vi "Cipher.vi"(5 "Key(input)":u32[](array[numeric])=[64, 226, 1, 0, 21, 21, 21, 21, 0, 0, 0, 0, 0, 0, 0, 0], 9 "ExpandedKey(w)1D":u32[](array[numeric]), 11 "error in":errorcluster) -> (8 "Cypher Output":u16[](array[numeric]), 15 "error out":errorcluster)   [LabVIEW 2012, in "Advanced Encryption Standard (AES).lvlib"]
doc: "The AES cipher is specified as a number of repetitions of transformation rounds that convert the input plaintext into the final output of ciphertext. Each round consists of several processing steps, including one that depends on the encryption key.\n\n<inline>"
uses:
  Advanced Encryption Standard (AES).lvlib
  Controls and Typedefs/Cipher Phases Enum (Typedef).ctl
panel:
  in  "Nb":i32=4
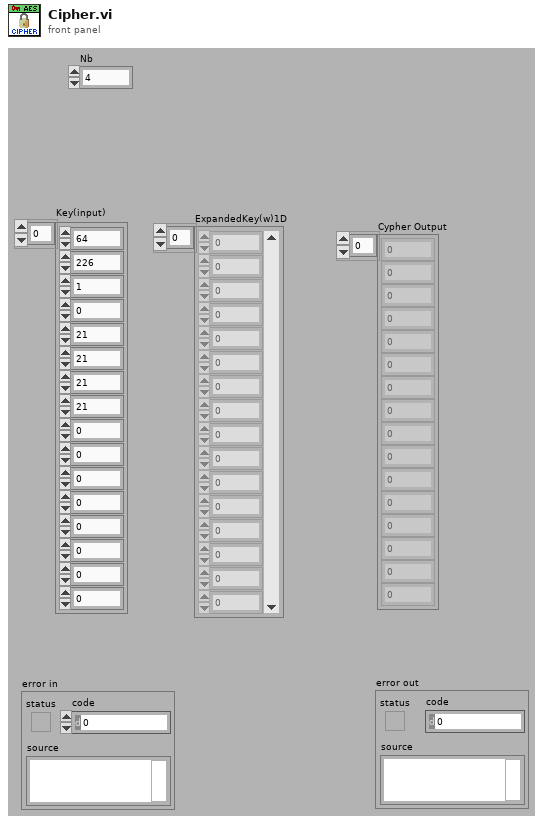
[diagram p1: front panel]
types:
  T1 = typedef "Cipher Phases Enum (Typedef).ctl" = enum16{"Init", "Mix rows"}
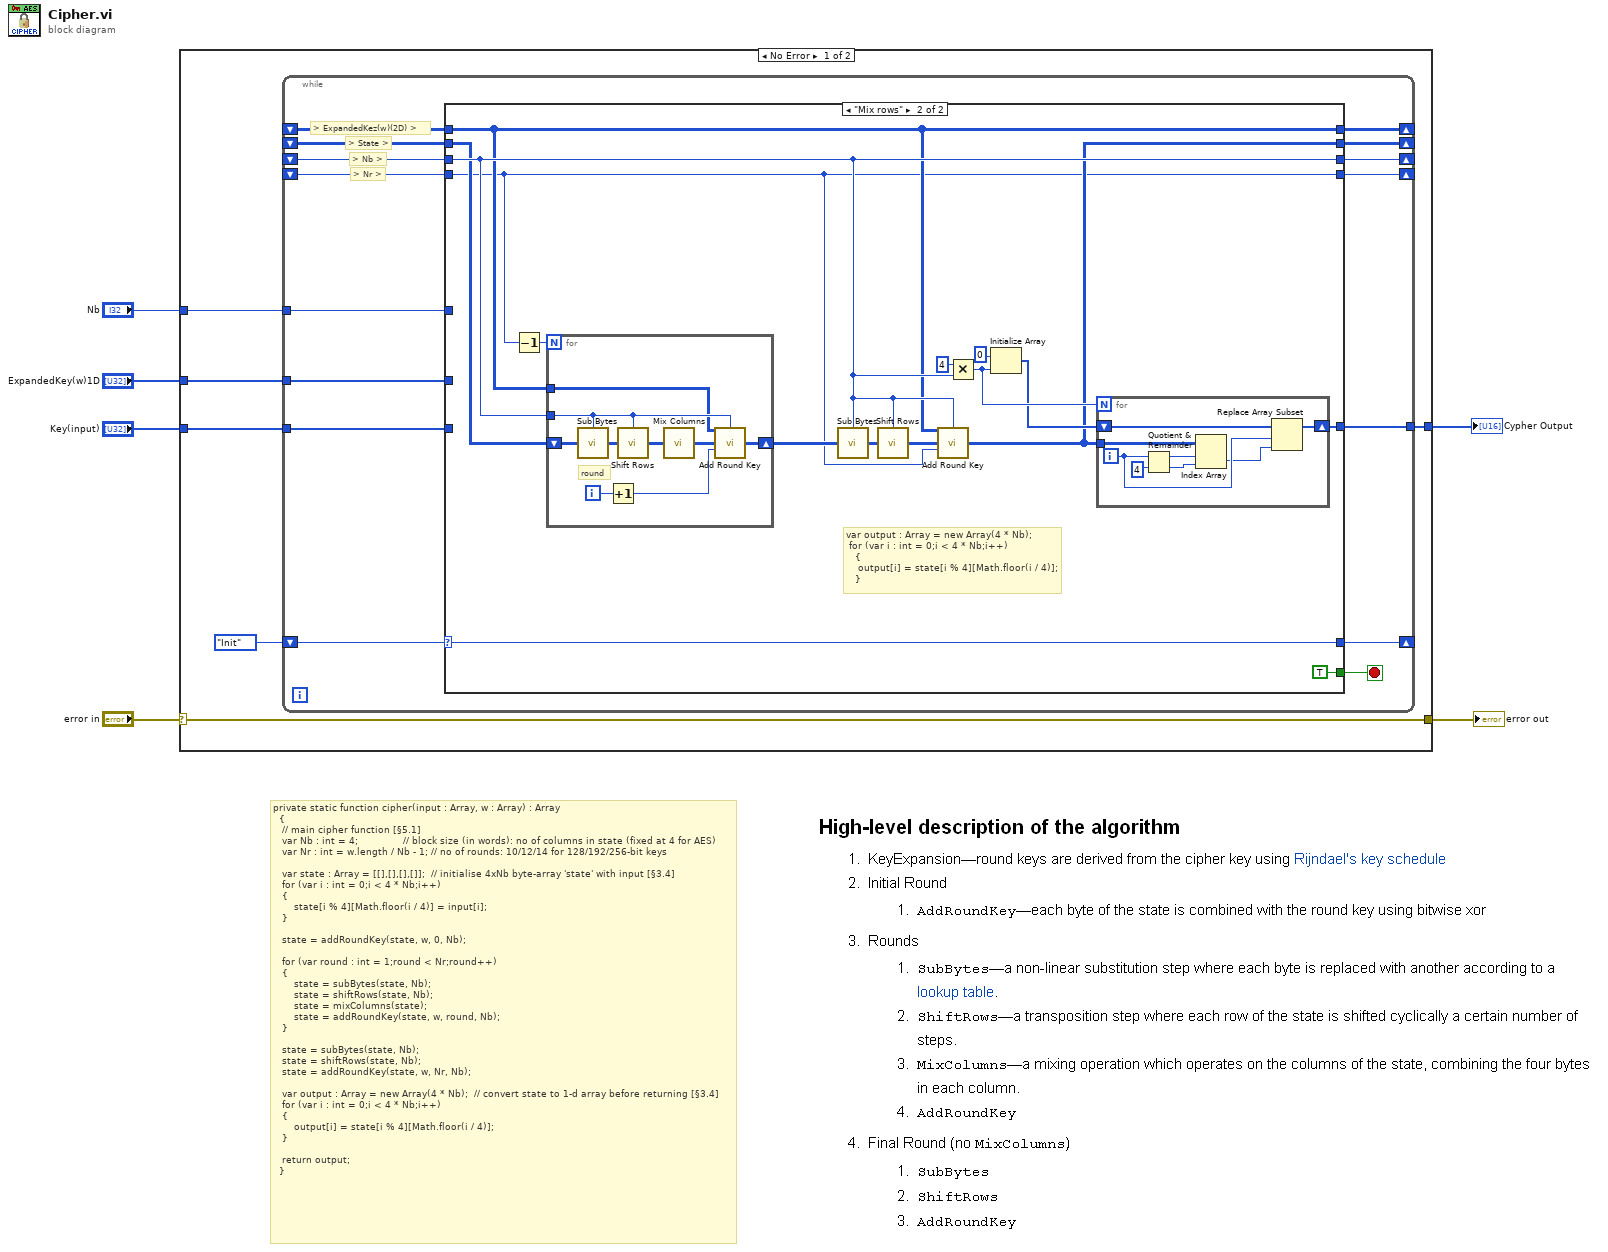
[diagram p0: block diagram]
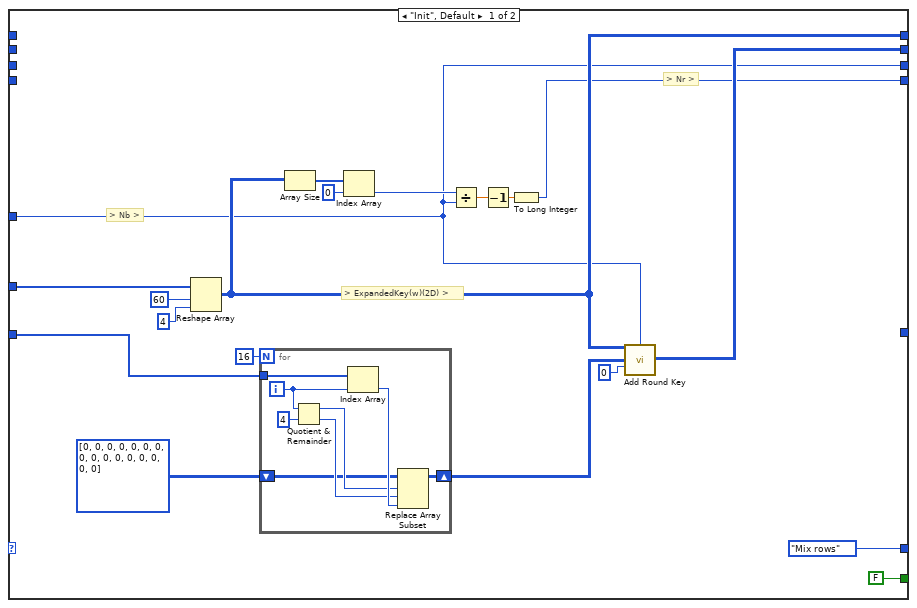
[diagram p2: hidden frame]
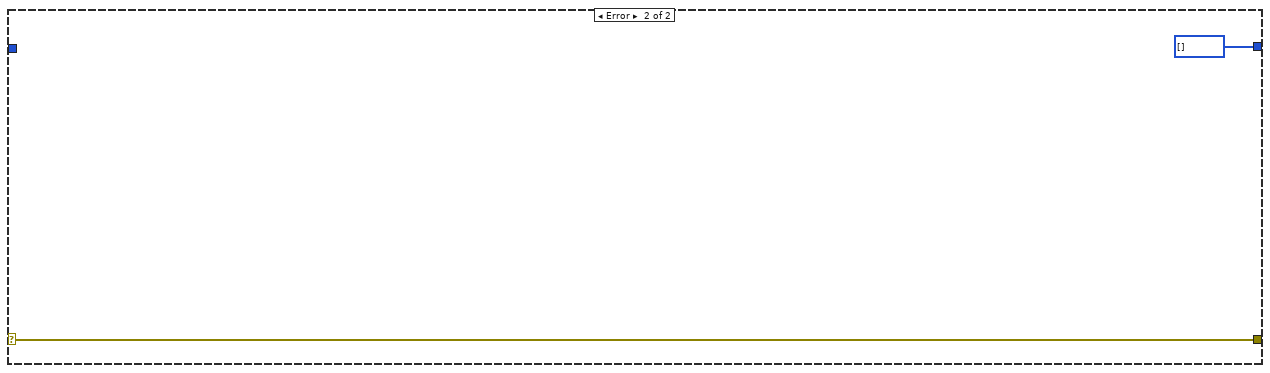
[diagram p3: hidden frame]
diagram:
  # "private static function cipher(input : Array, w : Array) : Array \n\t\t{    \n\t\t\t// main cipher function [§5.1]\n\t\t\tvar Nb : int = 4;               // block size (in words): no of columns in state (fixed at 4 for AES)\n\t\t\tvar Nr : int = w.length / Nb - 1; // no of rounds: 10/12/14 for 128/192/256-bit keys\n\n\t\t\tvar state : Array = [[],[],[],[]];  // initialise 4xNb byte-array 'state' with input [§3.4]\n\t\t\tfor (var i : int = 0;i < 4 * Nb;i++) \n\t\t\t{\n\t\t\t\t   state[i % 4][Math.floor(i / 4)] = input[i];\n\t\t\t}\n\t\t\t\n\t\t\tstate = addRoundKey(state, w, 0, Nb);\n\t\t\t\n\t\t\tfor (var round : int = 1;round < Nr;round++) \n\t\t\t{\n\t\t\t   \tstate = subBytes(state, Nb);\n\t\t   \t\tstate = shiftRows(state, Nb);\n\t\t   \t\tstate = mixColumns(state);\n\t\t   \t\tstate = addRoundKey(state, w, round, Nb);\n\t\t\t}\n\t\t\t\n\t\t\tstate = subBytes(state, Nb);\n\t\t\tstate = shiftRows(state, Nb);\n\t\t\tstate = addRoundKey(state, w, Nr, Nb);\n\t\t\t\n\t\t\tvar output : Array = new Array(4 * Nb);  // convert state to 1-d array before returning [§3.4]\n\t\t\tfor (var i : int = 0;i < 4 * Nb;i++)\n   {\n       output[i] = state[i % 4][Math.floor(i / 4)];\n\t\t\t}\n\n\t\t\treturn output;\n\t\t}"
  n1 = case shown="No Error" "error in" {
    selector: "error in" -> [w7 w89]
    tunnel: [w7 w89] -> w5
    tunnel: "ExpandedKey(w)1D" -> [w11 _]
    tunnel: "Key(input)" -> [w10 _]
    tunnel: [w9 u16[] []] -> w2
    tunnel: "Nb" -> [w8 _]
    frame No Error {
      n2 = while {
        shift-right: [w15] -> _
        shift-left: Cipher_Phases_Enum_(Typedef)."Init" ("Cipher Phases") -> [w27]
        tunnel: w11 -> [w26]
        tunnel: w10 -> [w25]
        shift-right: [w24] -> _
        shift-left: _ -> [w23]
        shift-right: [w22] -> _
        shift-left: _ -> [w21]
        shift-right: [w20] -> _
        shift-left: _ -> [w19]
        shift-right: [w18] -> _
        shift-left: _ -> [w17]
        tunnel: [w16] -> w9
        tunnel: w8 -> [w13]
        stop <- w14 stop-if-true
        # "> Nr >"
        # "> Nb >"
        # "> State >"
        # "> ExpandedKez(w)(2D) >"
        n3 = case shown="\"Mix rows\"" w27 {
          selector: w27 -> [_ w55]
          tunnel: w26 -> [w40 _]
          tunnel: w25 -> [w38 _]
          tunnel: [w36 w63] -> w24
          tunnel: w23 -> [_ w63]
          tunnel: [w35 w57] -> w22
          tunnel: w21 -> [_ w58]
          tunnel: [w30 w64] -> w20
          tunnel: w19 -> [_ w64]
          tunnel: [w33 w56] -> w18
          tunnel: w17 -> [_ w56]
          tunnel: [_ w60] -> w16
          tunnel: [Cipher_Phases_Enum_(Typedef)."Mix rows" ("Cipher Phases") w55] -> w15
          tunnel: [FALSE TRUE] -> w14
          tunnel: w13 -> [w30 _]
          frame "Init", Default {
            # "> Nb >"
            # "> ExpandedKey(w)(2D) >"
            # "> Nr >"
            n4 = Reshape Array(w40, 60 ("dimension size"), 4 ("dimension size")) -> (w36:u32[][])
            n5 = for {
              N: 16 -> [_]
              tunnel: w38 -> [w50]
              shift-right: [w48] -> w37
              shift-left: u16[][] [[0, 0, 0, 0], [0, 0, 0, 0], [0, 0, 0, 0], [0, 0, 0, 0]] ("State.Out") -> [w49]
              i -> [w47]
              n6 = Quotient & Remainder(x=w47, y=4) -> (x-y*floor(x/y)=w52:i32, floor(x/y)=w51:i32)
              n7 = Index Array(array=w50, index=w47) -> (element=w53:u32)
              n8 = Replace Array Subset(array=w49, new element=w53, index (row)=w52, index (col)=w51) -> (w48:u16[][])
            }
            n9 = Array Size(array=w36) -> (size(s)=w41:i32[])
            n10 = Index Array(array=w41, index=0) -> (element=w44:i32)
            n11 = Divide(x=w44, y=w30) -> (x/y=w43:dbl)
            n12 = Decrement(x=w43) -> (x-1=w34:dbl)
            n13 = To Long Integer(number=w34) -> (32bit integer=w33:i32)
            n14 = call "Add Round Key.vi"("ExpandedKey(w)"=w36, "Nb"=w30, "State.In"=w37, "rnd (0)"=0) -> ("State.Out"=w35:u16[][])  [unwired: 10 in, 1 out]
          }
          frame "Mix rows" {
            # "var output : Array = new Array(4 * Nb); \n\tfor (var i : int = 0;i < 4 * Nb;i++)\n   {\n    output[i] = state[i % 4][Math.floor(i / 4)];\n\t\t\t}"
            n15 = Decrement(x=w56) -> (x-1=w70:i32)
            n16 = for {
              N: w70 -> [_]
              shift-right: [w82] -> w65
              shift-left: w58 -> [w83]
              tunnel: w64 -> [w81]
              tunnel: w63 -> [w80]
              i -> [w84]
              # "round"
              n17 = call "Sub Bytes.vi"("Nb"=w81, "State In"=w83) -> ("State Out"=w87:u16[][])  [unwired: 12 in, 1 out]
              n18 = Increment(x=w84) -> (x+1=w79:i32)
              n19 = call "Shift Rows.vi"("Nb"=w81, "State In"=w87) -> ("State Out"=w86:u16[][])  [unwired: 12 in, 1 out]
              n20 = call "Mix Columns.vi"("State In"=w86) -> ("State Out"=w85:u16[][])  [unwired: 13 in, 1 out]
              n21 = call "Add Round Key.vi"("ExpandedKey(w)"=w80, "Nb"=w81, "State.In"=w85, "rnd (0)"=w79) -> ("State.Out"=w82:u16[][])  [unwired: 10 in, 1 out]
            }
            n22 = call "Sub Bytes.vi"("Nb"=w64, "State In"=w65) -> ("State Out"=w69:u16[][])  [unwired: 12 in, 1 out]
            n23 = call "Shift Rows.vi"("Nb"=w64, "State In"=w69) -> ("State Out"=w68:u16[][])  [unwired: 12 in, 1 out]
            n24 = call "Add Round Key.vi"("ExpandedKey(w)"=w63, "Nb"=w64, "State.In"=w68, "rnd (0)"=w56) -> ("State.Out"=w57:u16[][])  [unwired: 10 in, 1 out]
            n25 = Multiply(x=4, y=w64) -> (x*y=w62:i32)
            n26 = Initialize Array(u16 0 ("x"), w62) -> (w61:u16[])
            n27 = for {
              N: w62 -> [_]
              shift-right: [w71] -> w60
              shift-left: w61 -> [w72]
              tunnel: w57 -> [w73]
              i -> [w75]
              n28 = Quotient & Remainder(x=w75, y=4) -> (x-y*floor(x/y)=w77:i32, floor(x/y)=w76:i32)
              n29 = Index Array(array=w73, index (row)=w77, index (col)=w76) -> (element=w74:u16)
              n30 = Replace Array Subset(array=w72, new element=w74, index=w75) -> (w71:u16[])
            }
          }
        }
      }
    }
    frame Error {
    }
  }
  "error out" <- w5
  "Cypher Output" <- w2
